vi "Curtin1_DeleteBadRun.vi"(9 "Settings":T1={"Name of test"="", "Date"=timestamp(0 s since 1904-01-01), "Location"="", "Template"="", "Soundcard"="", "resolution"=0, "Sampling rate"=0, "Ch1 Gain "=0.0, "Ch2 Gain"=0.0, "Sample time (s)"=0.0, "Pre-trigger (s)"=0.0, "Hammer Threshold"=0.0, "Positions"=0, "Taps/Position"=0, "Set Names"="", "Freq resolution"=0.0, "Hammer cutoff"=0.0, "Mic cutoff"=0.0, "Double bounce "=0.0, "Hammer Cal"=0.0, "dB Offset"=0.0, "Accel Cal"=0.0, "Vibrometer Cal"=0.0, "Mic Cal"=0.0, "Output"=0, "Voltage Cal"=0.0, "Vibrometer Port"="ASRL27::INSTR", "Range"=4, "High Pass"=2, "Bandwidth"=4, "X Range"=[], "Y Range"=[], "dB Spread"=0.0, "Trigger"=0, "Ch_1"=1, "Ch_2"=2, "flip?"=FALSE, "60Hz"=FALSE, "Time offset"=0.0, "Piezo Cal"=1.0, "Default Notes"=""} {"Ch_2" min=1 step=1; "Ch_1" min=1 max=100 step=1; "Trigger" items=["Hammer (force)", "Self-tap", "Spacebar"]; "Bandwidth" items=["1 kHz"=1, "5 kHz"=5, "10 kHz"=10, "25 kHz"=25, "50 kHz"=50, "100 kHz"=100]; "High Pass" items=["Off", "13 Hz", "104 Hz"]; "Range" items=["10 mm/s"=1, "20 mm/s"=2, "50 mm/s"=5, "100 mm/s"=10, "200 mm/s"=20, "500 mm/s"=50, "1 m/s"=100, "2 m/s"=200]; "Output" items=["Accelerometer", "Speed (from acceleration)", "Microphone", "Vibrometer", "Piezo"]; "Voltage Cal" format="%#_13g"; "Ch2 Gain" format="%#_13g"; "Ch1 Gain" format="%#_13g"; "Double bounce" min=0.0; "Mic cutoff" min=0.0 format="%#_4g"; "Hammer cutoff" min=0.0 format="%#_4g"; "Freq resolution" min=0.0; "Pre-trigger (s)" format="%#_13g"; "Date" format="%<%H:%M\n%d/%m/%y>T"; "resolution" items=["16 bit"=16, "24 bit"=24, "32 bit"=32]; "Sampling rate" items=["22050 samp/s"=22050, "44100 samp/s"=44100, "48000 samp/s"=48000]}, 10 "Last":path, 11 "Queue in":refnum<queue>) -> (3 "Last Data Set":path)   [LabVIEW 2024]
uses:
  PreferencesControl.ctl
  Mic/Mic_Global.vi
panel:
  # "Hz"
  # "dB"
  # "dB"
  # "sec"
  # "sec"
  # "mV/Pa"
  # "mV/m/s2"
  # "mV/mm/s"
  # "V/N"
  # "sec"
  # "sec"
  # "mV/N"
  # "a.u."
  # "a.u."
  # "sec"
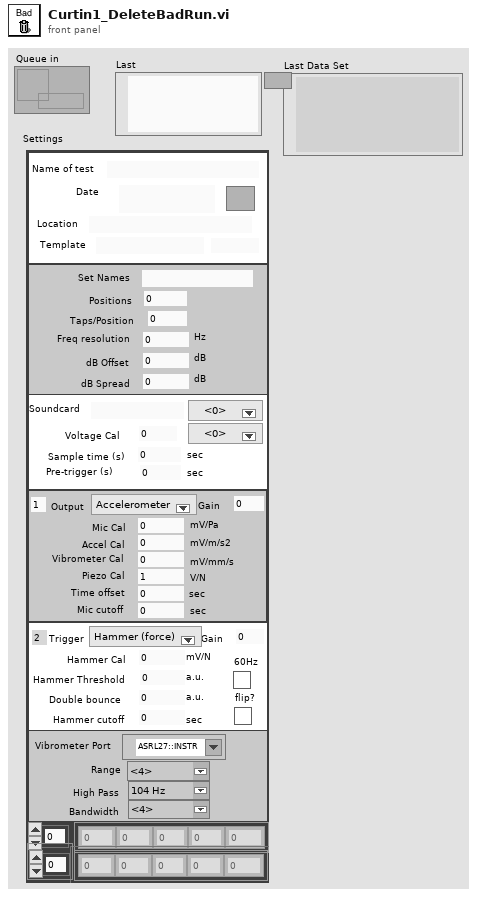
[diagram p1: front panel]
types:
  T1 = typedef "PreferencesControl.ctl" = cluster{"Name of test":string, "Date":timestamp, "Location":string, "Template":string, "Soundcard":string, "resolution":u16, "Sampling rate":u16, "Ch1 Gain ":dbl, "Ch2 Gain":dbl, "Sample time (s)":dbl, "Pre-trigger (s)":dbl, "Hammer Threshold":dbl, "Positions":i16, "Taps/Position":i16, "Set Names":string, "Freq resolution":dbl, "Hammer cutoff":dbl, "Mic cutoff":dbl, "Double bounce ":dbl, "Hammer Cal":dbl, "dB Offset":dbl, "Accel Cal":dbl, "Vibrometer Cal":dbl, "Mic Cal":dbl, "Output":u16, "Voltage Cal":dbl, "Vibrometer Port":refnum<visa-resource-name>, "Range":u16, "High Pass":u16, "Bandwidth":u16, "X Range":cluster{"Minimum":dbl, "Maximum":dbl, "Increment":dbl, "Minor Increment":dbl, "Start":dbl}[], "Y Range":cluster{"Minimum":dbl, "Maximum":dbl, "Increment":dbl, "Minor Increment":dbl, "Start":dbl}[], "dB Spread":dbl, "Trigger":u16, "Ch_1":u8, "Ch_2":u8, "flip?":bool, "60Hz":bool, "Time offset":dbl, "Piezo Cal":dbl, "Default Notes":string}
  T2 = enum16{"Initialize", "Free run", "One Shot - waiting", "One Shot - triggered", "Wait", "Close"}
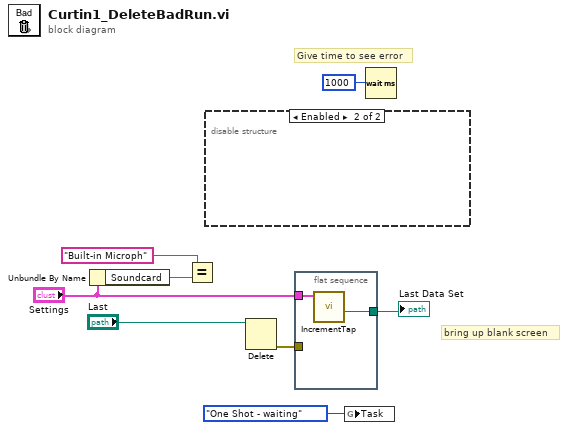
[diagram p0: block diagram]
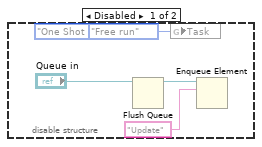
[diagram p2: hidden frame]
diagram:
  # "bring up blank screen"
  # "Give time to see error"
  n1 = Unbundle By Name("Settings") -> ("Soundcard"=w5:string)
  n2 = Equal?(x="Built-in Microph", y=w5) -> ()  [unwired: 1 out]
  n3 = disable-structure shown="Enabled" {
    frame Disabled {
      n4 = Flush Queue(queue="Queue in") -> (queue out=w13:refnum<queue>)  [unwired: 1 in, 2 out]
      n5 = global write "Mic_Global.vi" "Task"(T2."One Shot - waiting" ("Task")) -> ()
      n6 = global write "Mic_Global.vi" "Task"(T2."Free run" ("Task")) -> ()
      n7 = Enqueue Element(queue=w13, element="Update") -> ()  [unwired: 2 in, 3 out]
    }
    frame Enabled {
    }
  }
  n8 = Delete(path (use dialog)="Last") -> (error out=w2:errorcluster)  [unwired: 4 in, 2 out]
  n9 = flat-sequence {
    tunnel: "Settings" -> [w14]
    tunnel: [w15] -> w3
    tunnel: w2 -> [_]
    frame #0 {
      n10 = call "IncrementTap.vi"("Settings"=w14) -> ("Last Data Set"=w15:path)  [unwired: 5 in, 5 out]
    }
  }
  n11 = global write "Mic_Global.vi" "Task"(T2."One Shot - waiting" ("Task")) -> ()
  n12 = Wait (ms)(milliseconds to wait=u32 1000) -> ()  [unwired: 1 out]
  "Last Data Set" <- w3
